vi "FTW-Actor.vi"(0 "Actor Template-Core":refnum<class "Actor Template-Core.lvclass">, 5 "FTW Actor Instance Configuration":string="{\n  \"Identity\": \"ActorName\",\n  \"InboxAddress\": \"inproc://*\",\n  \"LoggerAddress\": \"\",\n  \"My Data\": false,\n  \"Publisher URI\": \"inproc://*\",\n  \"Subscriber URIs\": \"\",\n  \"Refresh Period\": 2\n}", 11 "ErrorIn":errorcluster) -> (15 "Error":errorcluster)   [LabVIEW 2015, in "Actor Template-Core.lvclass"]
uses:
  Actor Template-Core.lvclass
  source/actor/Message/Base/FTW-Message.lvclass
  Actor Template-Core.lvclass/Actor Template-Core.ctl
  source/actor/Instance/FTW-ActorInstance.lvclass/FTW-ActorInstance.ctl
  source/actor/JobSequencer/FTW-SEQ-Current.vi
  source/actor/Connector/FTW-ActorConnector.lvclass
  source/actor/Instance/FTW-ActorInstance.lvclass
  source/actor/Message/Request/FTW-Message-IncomingRequest.lvclass
  source/actor/Publisher/FTW-Publisher.lvclass
  source/actor/Subscriber/FTW-Subscriber.lvclass
panel:
  # "#TODO\nhide controls for a GUI"
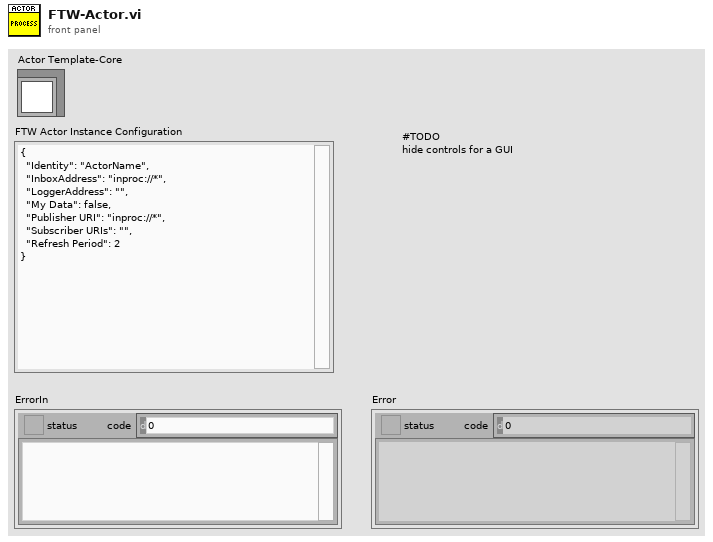
[diagram p1: front panel]
types:
  T1 = cluster{"Incoming Requests":refnum<event-registration>, "Local Messages":refnum<event-registration>, "Subscription":refnum<event-registration>}
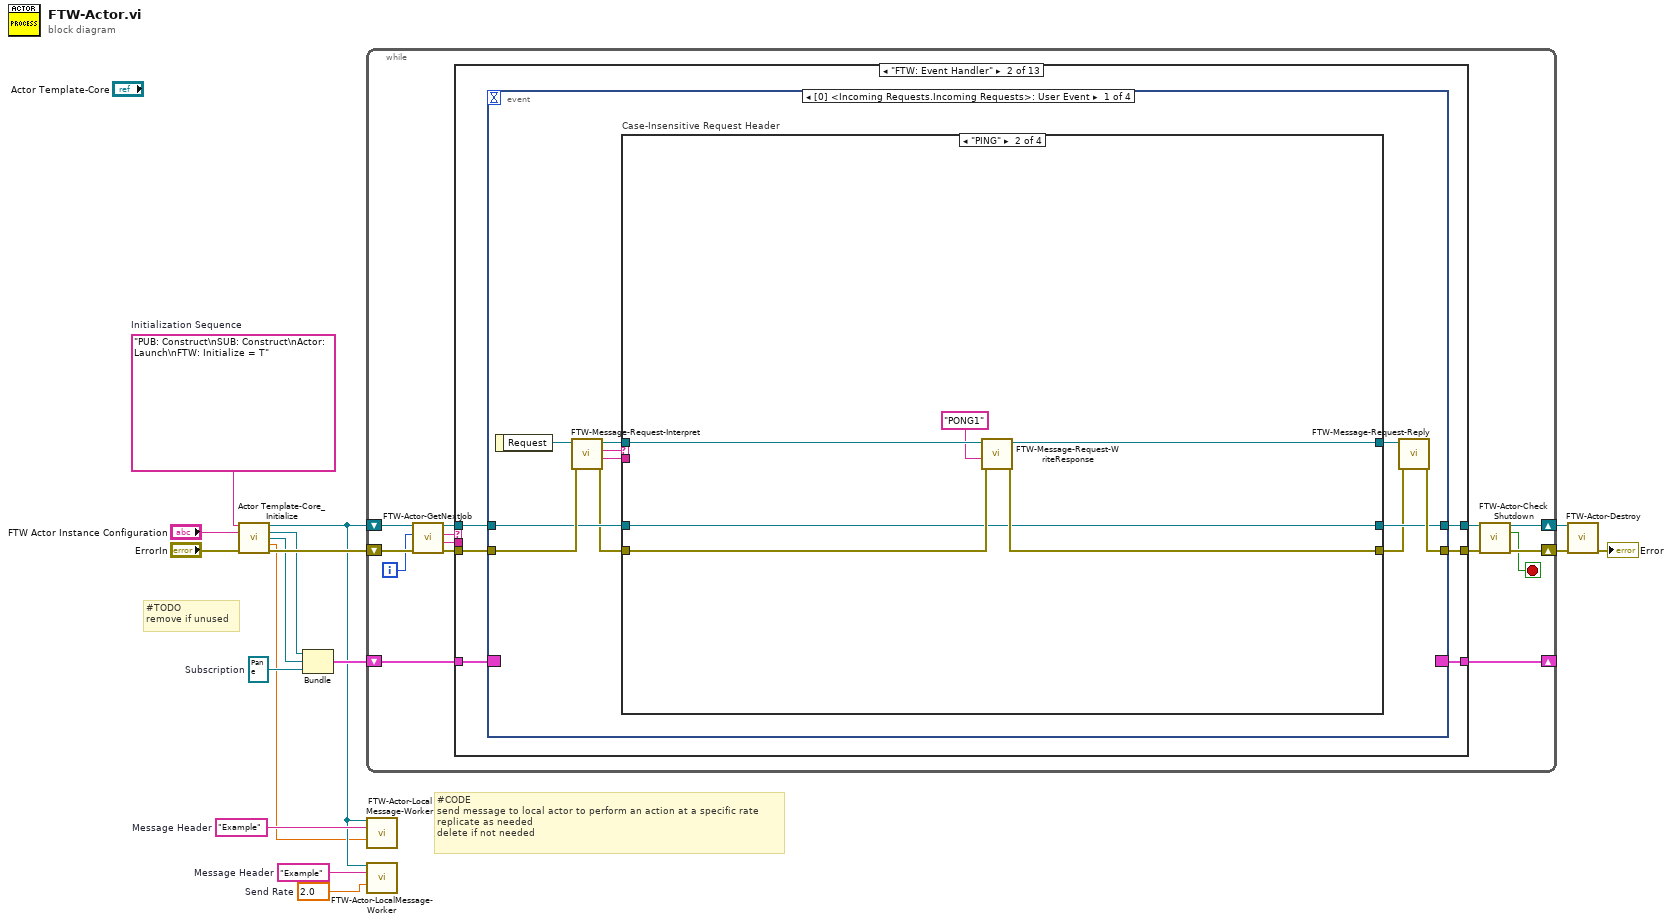
[diagram p0: block diagram]
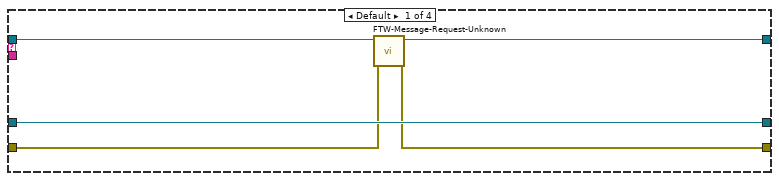
[diagram p3: hidden frame]
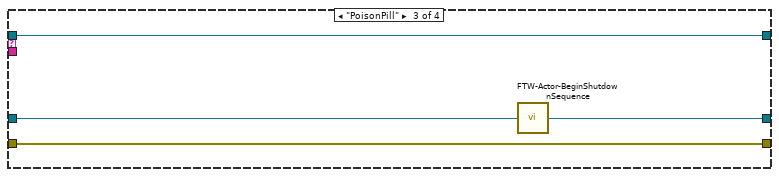
[diagram p4: hidden frame]
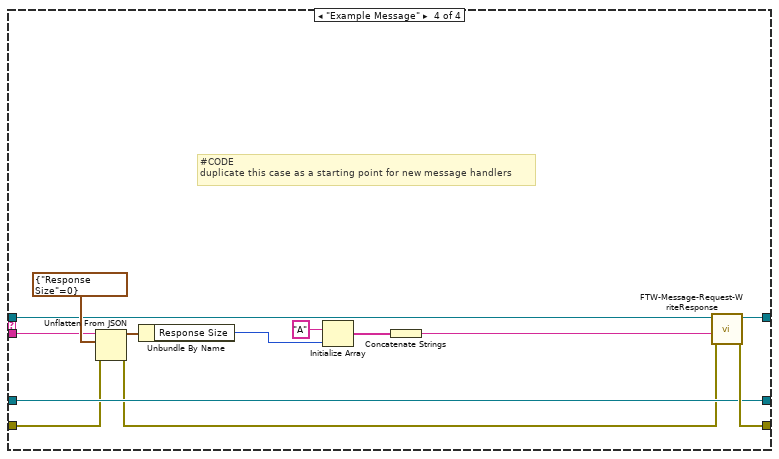
[diagram p5: hidden frame]
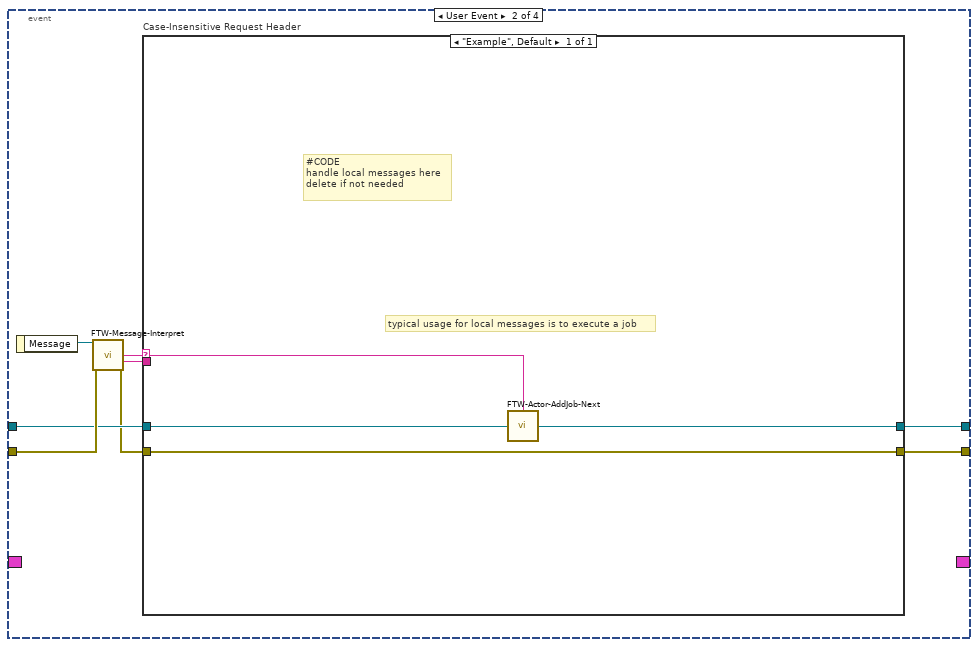
[diagram p6: hidden frame]
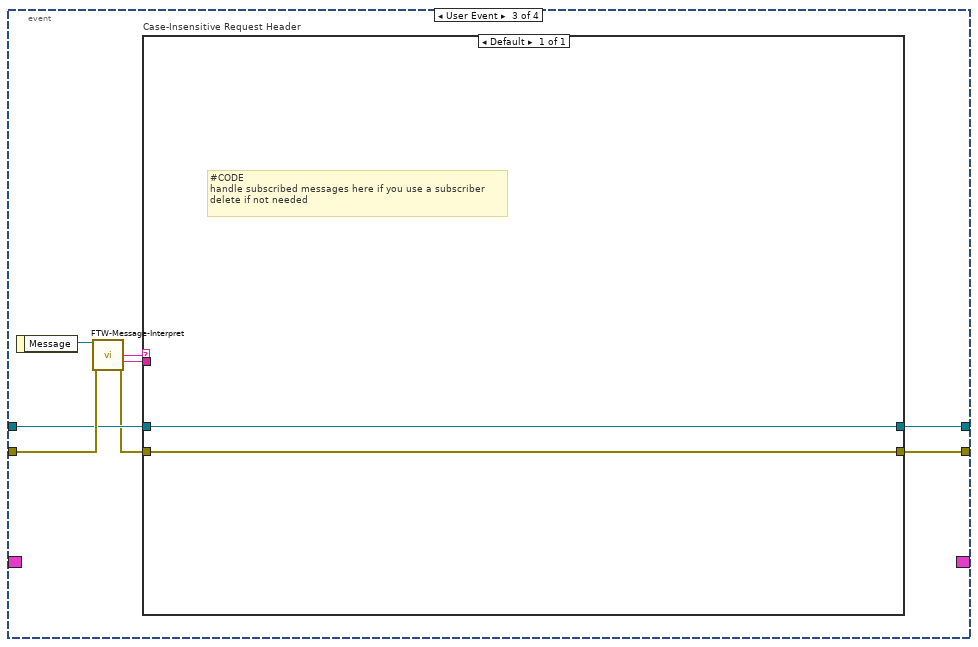
[diagram p7: hidden frame]
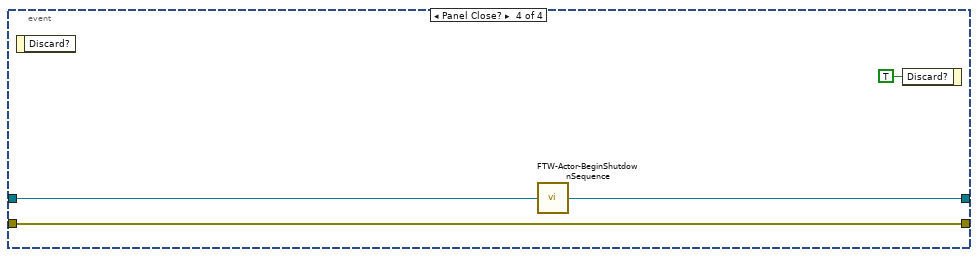
[diagram p8: hidden frame]
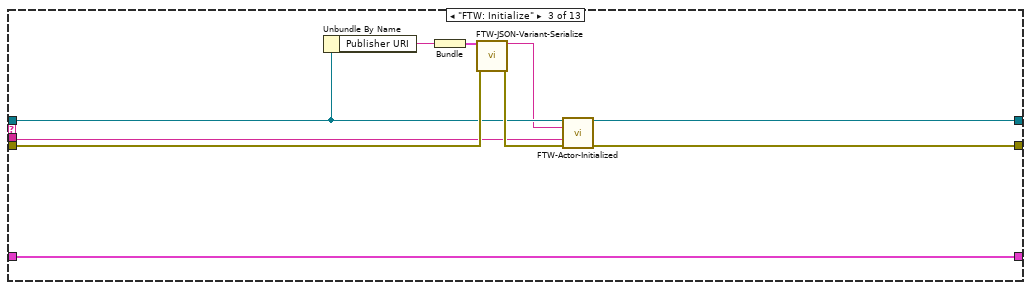
[diagram p9: hidden frame]
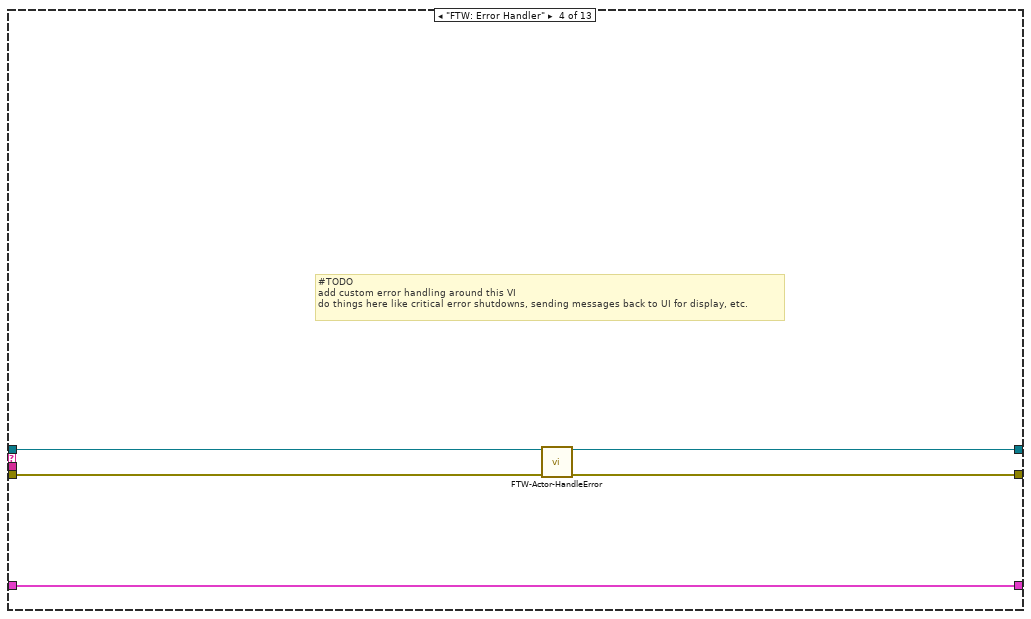
[diagram p10: hidden frame]
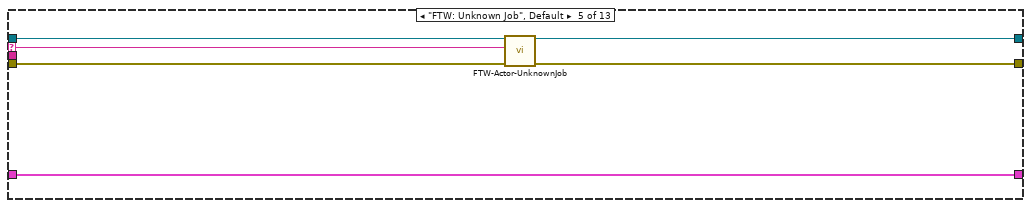
[diagram p11: hidden frame]
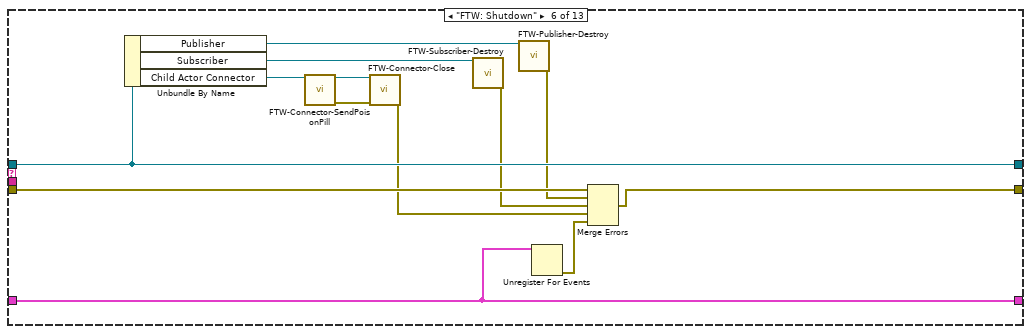
[diagram p12: hidden frame]
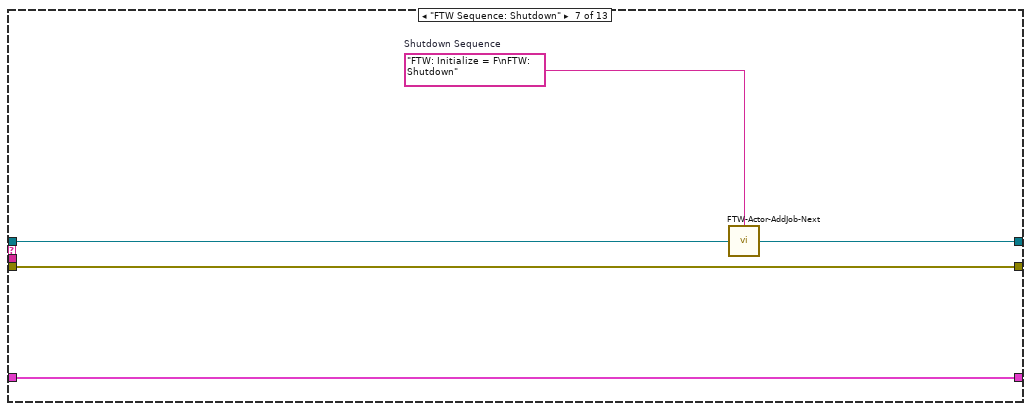
[diagram p13: hidden frame]
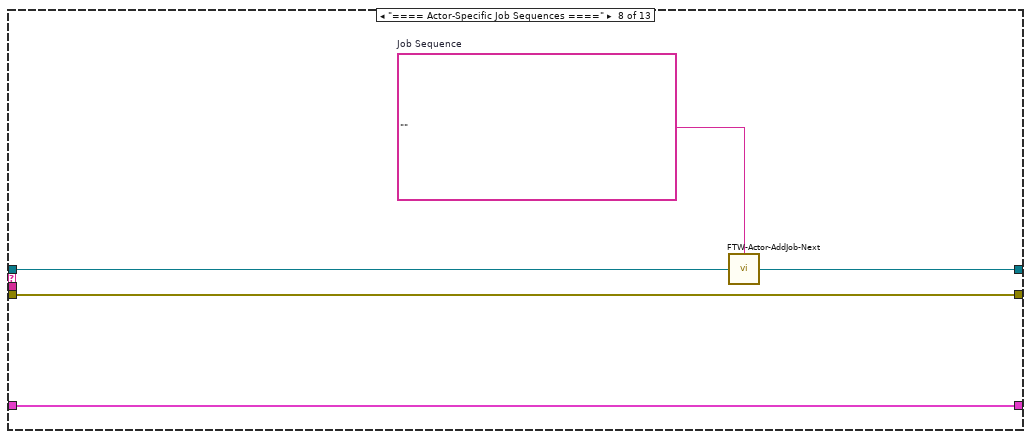
[diagram p14: hidden frame]
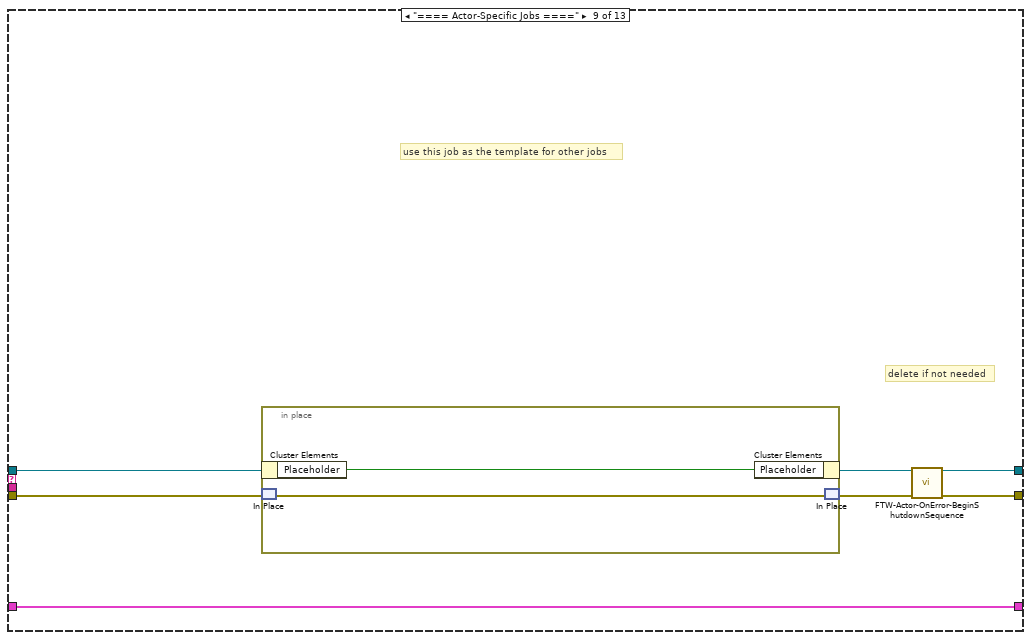
[diagram p15: hidden frame]
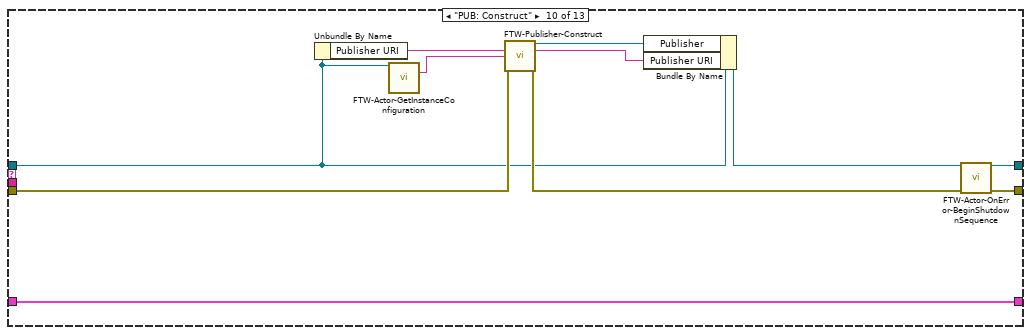
[diagram p16: hidden frame]
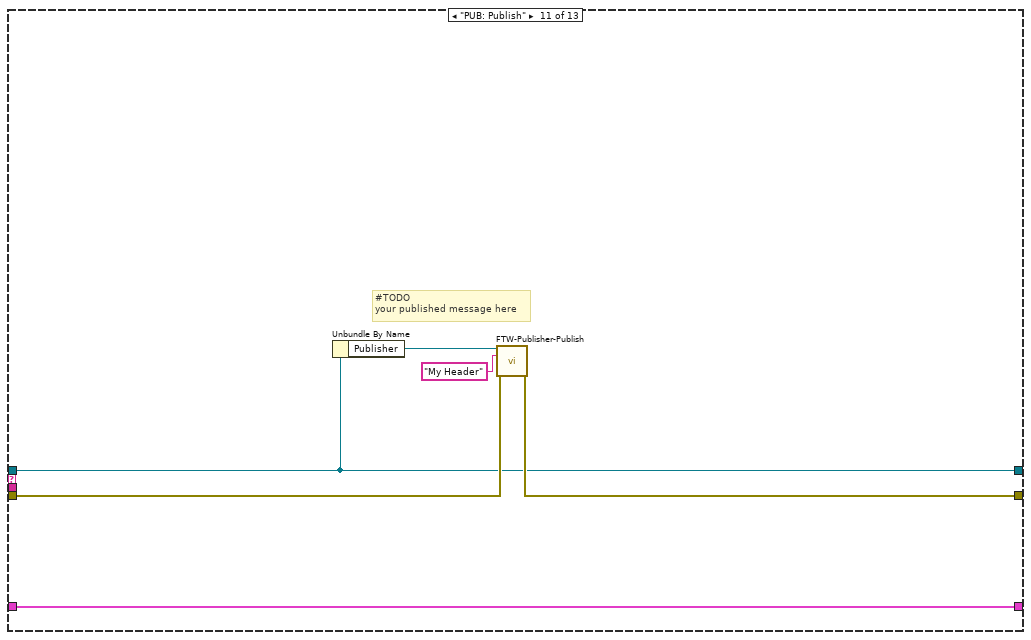
[diagram p17: hidden frame]
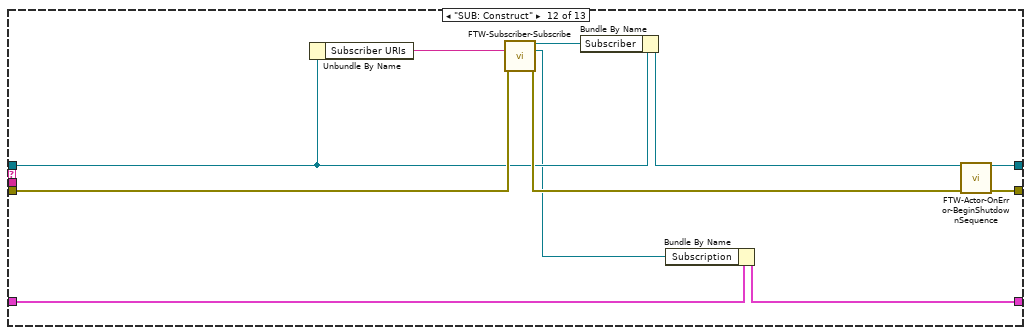
[diagram p18: hidden frame]
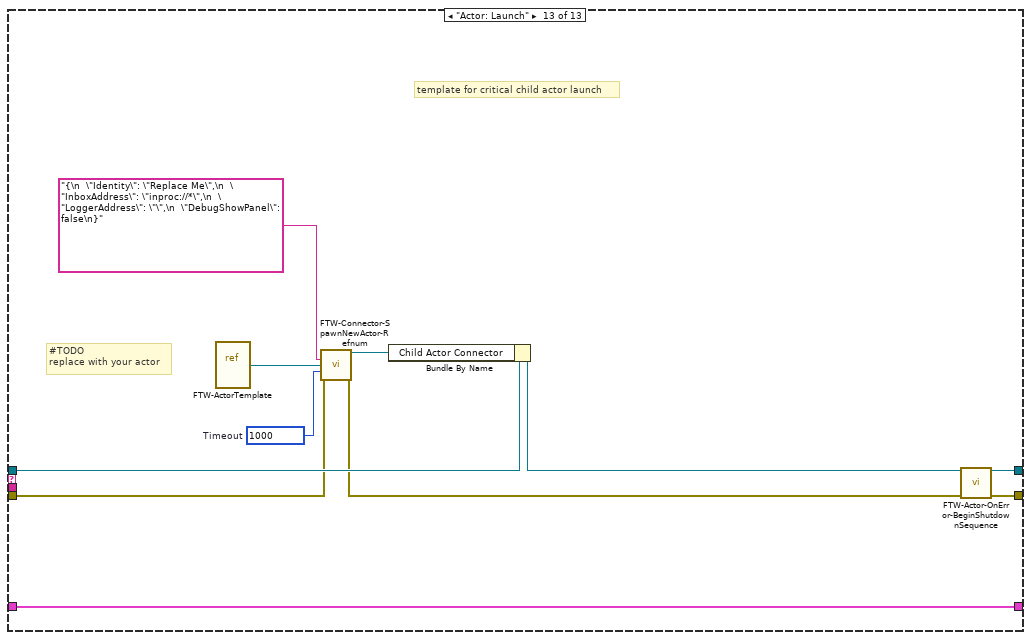
[diagram p19: hidden frame]
diagram:
  w4 = 2.0  # Send Rate
  w3 = "Example"  # Message Header
  w5 = "Example"  # Message Header
  w6 = refnum<event-registration> refnum  # Subscription
  w12 = "PUB: Construct\nSUB: Construct\nActor: Launch\nFTW: Initialize = T"  # Initialization Sequence
  # "#CODE\nsend message to local actor to perform an action at a specific rate\nreplicate as needed\ndelete if not needed"
  # "#TODO\nremove if unused"
  n1 = call "Actor Template-Core_Initialize.vi"("Initialization Sequence"=w12, "FTW Actor Instance Configuration"="FTW Actor Instance Configuration", "error in (no error)"="ErrorIn") -> ("Actor Template-Core out"=w2:refnum<class "Actor Template-Core.lvclass">, "Incoming Requests"=w8:refnum<event-registration>, "Local Messages"=w7:refnum<event-registration>, "Refresh Period"=w1:dbl, "error out"=w13:errorcluster)  [unwired: 8 in]
  n2 = Bundle("Incoming Requests"=w8, "Local Messages"=w7, "Subscription"=w6) -> (w10:T1)  [unwired: 1 in]
  n3 = while {
    shift-right: [w20] -> w15
    shift-left: w13 -> [w27]
    shift-right: [w17] -> _
    shift-left: w10 -> [w30]
    shift-right: [w22] -> w16
    shift-left: w2 -> [w29]
    i -> [w18]
    stop <- w19 stop-if-true
    n4 = call "FTW-Actor-GetNextJob.vi"("error in"=w27, "Jobs Performed"=w18, "FTW Actor Instance"=w29) -> ("error out"=w26:errorcluster, "Job Data"=w24:string, "Job Name"=w25:string, "FTW Actor Instance out"=w28:refnum<class "Actor Template-Core.lvclass">)  [unwired: 5 in]
    n5 = case shown="\"FTW: Event Handler\"" w25 {
      selector: w25 -> [_ _ _ _ w120 _ _ _ _ _ _ _ _]
      tunnel: [w32 w39 w110 w115 w123 w137 w142 w147 w151 w164 w172 w181 w195] -> w21
      tunnel: w26 -> [w32 w38 w114 w117 w124 w138 w142 w147 w154 w166 w173 w183 w189]
      tunnel: w30 -> [w33 w34 w112 w119 w125 w135 w143 w148 w155 w168 w174 w185 w196]
      tunnel: [w33 w37 w112 w119 w125 w135 w143 w148 w155 w168 w174 w176 w196] -> w17
      tunnel: w24 -> [_ _ w107 _ _ _ _ _ _ _ _ _ _]
      tunnel: [w31 w36 w111 w116 w121 w134 w140 w145 w149 w162 w171 w179 w194] -> w23
      tunnel: w28 -> [w31 w35 w109 w118 w122 w134 w141 w146 w152 w159 w171 w177 w193]
      frame "==== Featherweight Framework Jobs ====" {
      }
      frame "FTW: Event Handler" {
        n6 = event shown="[0] <Incoming Requests.Incoming Requests>: User Event" {
          selector: w34 -> [_ _ _ _]
          dyn-events: [_ _ _ _] -> w37
          timeout: _ -> [_ _ _ _]
          tunnel: [w49 w81 w93 w103] -> w39
          tunnel: w38 -> [w48 w85 w97 w103]
          tunnel: [w43 w82 w94 w101] -> w36
          tunnel: w35 -> [w47 w84 w96 w102]
          event User Event {
            n7 = event-data() -> ("Request"=w50:refnum<class "FTW-Message-IncomingRequest.lvclass">)  [unwired: 1 in]
            n8 = call "FTW-Message-Request-Interpret.vi"("error in"=w48, "FTW Incoming Request"=w50) -> ("error out"=w46:errorcluster, "Request Body"=w40:string, "Request Header"=w44:string, "FTW Incoming Request out"=w45:refnum<class "FTW-Message-IncomingRequest.lvclass">)  [unwired: 6 in]
            n9 = case "Case-Insensitive Request Header" shown="\"PING\"" w44 {
              tunnel: [w53 w59 w64 w78] -> w42
              tunnel: w46 -> [w54 w60 w64 w67]
              tunnel: [w55 w58 w65 w76] -> w43
              tunnel: w47 -> [w55 w58 w63 w76]
              tunnel: w45 -> [w52 w61 w62 w68]
              tunnel: [w51 w57 w62 w77] -> w41
              tunnel: w40 -> [_ _ _ w66]
              frame Default {
                n10 = call "FTW-Message-Request-Unknown.vi"("error in"=w54, "FTW Incoming Request"=w52) -> ("error out"=w53:errorcluster, "FTW Incoming Request Out"=w51:refnum<class "FTW-Message-IncomingRequest.lvclass">)  [unwired: 8 in]
              }
              frame "PING" {
                n11 = call "FTW-Message-Request-WriteResponse.vi"("error in"=w60, "Response Body"="PONG1" ("Response Header"), "FTW Incoming Request"=w61) -> ("error out"=w59:errorcluster, "FTW Incoming Request out"=w57:refnum<class "FTW-Message-IncomingRequest.lvclass">)  [unwired: 7 in]
              }
              frame "PoisonPill" {
                n12 = call "FTW-Actor-BeginShutdownSequence.vi"("FTW Actor Instance"=w63) -> ("FTW Actor Instance out"=w65:refnum<class "Actor Template-Core.lvclass">)  [unwired: 3 in]
              }
              frame "Example Message" {
                # "#CODE\nduplicate this case as a starting point for new message handlers"
                n13 = Unflatten From JSON(JSON string=w66, type and defaults=cluster{"Response Size":i32} {"Response Size"=0}, error in (no error)=w67) -> (value=w73:cluster{"Response Size":i32}, error out=w75:errorcluster)  [unwired: 4 in]
                n14 = Unbundle By Name(w73) -> ("Response Size"=w72:i32)
                n15 = Initialize Array("A", w72) -> (w70:string[])
                n16 = Concatenate Strings(w70) -> (w69:string)
                n17 = call "FTW-Message-Request-WriteResponse.vi"("error in"=w75, "Response Body"=w69, "FTW Incoming Request"=w68) -> ("error out"=w78:errorcluster, "FTW Incoming Request out"=w77:refnum<class "FTW-Message-IncomingRequest.lvclass">)  [unwired: 7 in]
              }
            }
            n18 = call "FTW-Message-Request-Reply.vi"("FTW: Reply Error"=w42, "FTW Incoming Request"=w41) -> ("error out"=w49:errorcluster)  [unwired: 8 in, 1 out]
          }
          event User Event {
            n19 = event-data() -> ("Message"=w86:refnum<class "FTW-Message.lvclass">)  [unwired: 1 in]
            n20 = call-dynamic "FTW-Message-Interpret.vi"("FTW Message"=w86, "error in"=w85) -> ("Message Header"=w80:string, "Message Body"=w79:string, "error out"=w83:errorcluster)  [unwired: 9 in, 2 out]
            n21 = case "Case-Insensitive Request Header" shown="\"Example\", Default" w80 {
              selector: w80 -> [w87]
              tunnel: [w89] -> w81
              tunnel: w83 -> [w89]
              tunnel: [w88] -> w82
              tunnel: w84 -> [w90]
              tunnel: w79 -> [_]
              frame "Example", Default {
                # "#CODE\nhandle local messages here\ndelete if not needed"
                # "typical usage for local messages is to execute a job"
                n22 = call "FTW-Actor-AddJob-Next.vi"("Add Next in Job Queue"=w87, "FTW Actor Instance"=w90) -> ("FTW Actor Instance out"=w88:refnum<class "Actor Template-Core.lvclass">)  [unwired: 2 in]
              }
            }
          }
          event User Event {
            n23 = event-data() -> ("Message"=w98:refnum<class "FTW-Message.lvclass">)  [unwired: 1 in]
            n24 = call-dynamic "FTW-Message-Interpret.vi"("FTW Message"=w98, "error in"=w97) -> ("Message Header"=w92:string, "Message Body"=w91:string, "error out"=w95:errorcluster)  [unwired: 9 in, 2 out]
            n25 = case "Case-Insensitive Request Header" shown="Default" w92 {
              tunnel: [w99] -> w93
              tunnel: w95 -> [w99]
              tunnel: [w100] -> w94
              tunnel: w96 -> [w100]
              tunnel: w91 -> [_]
              frame Default {
                # "#CODE\nhandle subscribed messages here if you use a subscriber\ndelete if not needed"
              }
            }
          }
          event Panel Close? {
            n26 = event-data() -> ()  [unwired: 1 in, 1 out]
            n27 = call "FTW-Actor-BeginShutdownSequence.vi"("FTW Actor Instance"=w102) -> ("FTW Actor Instance out"=w101:refnum<class "Actor Template-Core.lvclass">)  [unwired: 3 in]
            n28 = event-data("Discard?"=TRUE) -> ()  [unwired: 1 in, 1 out]
          }
        }
      }
      frame "FTW: Initialize" {
        n29 = Unbundle By Name(w109) -> ("Publisher URI"=w108:string)
        n30 = Bundle("Publisher URI"=w108) -> (w106:cluster{"Publisher URI":string})  [unwired: 1 in]
        n31 = call "FTW-JSON-Variant-Serialize.vi"("Variant"=w106, "error in"=w114) -> ("JSON String"=w105:string, "error out"=w113:errorcluster)  [unwired: 12 in]
        n32 = call-dynamic "FTW-Actor-Initialized.vi"("FTW Actor Instance"=w109, "Initialized Response"=w105, "Positive Init?"=w107, "error in"=w113) -> ("FTW Actor Instance out"=w111:refnum<class "Actor Template-Core.lvclass">, "error out"=w110:errorcluster)  [unwired: 10 in]
      }
      frame "FTW: Error Handler" {
        # "#TODO\nadd custom error handling around this VI\ndo things here like critical error shutdowns, sending messages back to UI for display, etc."
        n33 = call-dynamic "FTW-Actor-HandleError.vi"("FTW Actor Instance"=w118, "error in"=w117) -> ("FTW Actor Instance out"=w116:refnum<class "Actor Template-Core.lvclass">, "error out"=w115:errorcluster)  [unwired: 10 in, 2 out]
      }
      frame "FTW: Unknown Job", Default {
        n34 = call-dynamic "FTW-Actor-UnknownJob.vi"("FTW Actor Instance"=w122, "Unknown Job"=w120, "error in"=w124) -> ("FTW Actor Instance out"=w121:refnum<class "Actor Template-Core.lvclass">, "error out"=w123:errorcluster)  [unwired: 11 in]
      }
      frame "FTW: Shutdown" {
        n35 = Unbundle By Name(w134) -> ("Publisher"=w133:refnum<class "FTW-Publisher.lvclass">, "Subscriber"=w131:refnum<class "FTW-Subscriber.lvclass">, "Child Actor Connector"=w129:refnum<class "FTW-ActorConnector.lvclass">)
        n36 = call-dynamic "FTW-Connector-SendPoisonPill.vi"("FTW Actor Connector"=w129) -> ("FTW Actor Connector out"=w128:refnum<class "FTW-ActorConnector.lvclass">, "error out"=w127:errorcluster)  [unwired: 9 in, 4 out]
        n37 = call-dynamic "FTW-Connector-Close.vi"("FTW Actor Connector"=w128, "error in"=w127) -> ("error out"=w126:errorcluster)  [unwired: 13 in]
        n38 = call "FTW-Subscriber-Destroy.vi"("FTW-Subscription In"=w131) -> ("error out"=w130:errorcluster)  [unwired: 14 in]
        n39 = call "FTW-Publisher-Destroy.vi"("FTW-Publisher In"=w133) -> ("error out"=w132:errorcluster)  [unwired: 14 in]
        n40 = Unregister For Events(event registration refnum=w135) -> (error out=w136:errorcluster)  [unwired: 1 in]
        n41 = Merge Errors(w138, w132, w130, w126, w136) -> (w137:errorcluster)
      }
      frame "FTW Sequence: Shutdown" {
        w139 = "FTW: Initialize = F\nFTW: Shutdown"  # Shutdown Sequence
        n42 = call "FTW-Actor-AddJob-Next.vi"("Add Next in Job Queue"=w139, "FTW Actor Instance"=w141) -> ("FTW Actor Instance out"=w140:refnum<class "Actor Template-Core.lvclass">)  [unwired: 2 in]
      }
      frame "==== Actor-Specific Job Sequences ====" {
        w144 = ""  # Job Sequence
        n43 = call "FTW-Actor-AddJob-Next.vi"("Add Next in Job Queue"=w144, "FTW Actor Instance"=w146) -> ("FTW Actor Instance out"=w145:refnum<class "Actor Template-Core.lvclass">)  [unwired: 2 in]
      }
      frame "==== Actor-Specific Jobs ====" {
        # "delete if not needed"
        # "use this job as the template for other jobs"
        n44 = in-place {
          n45 = in-place-cluster #1(w152) -> ("Placeholder"=w156:bool)
          n46 = in-place-match #2(w154) -> (w157:errorcluster)
          n47 = in-place-cluster #1("Placeholder"=w156) -> (w150:refnum<class "Actor Template-Core.lvclass">)
          n48 = in-place-match #2(w157) -> (w153:errorcluster)
        }
        n49 = call-dynamic "FTW-Actor-OnError-BeginShutdownSequence.vi"("FTW Actor Instance"=w150, "error in"=w153) -> ("FTW Actor Instance out"=w149:refnum<class "Actor Template-Core.lvclass">, "error out"=w151:errorcluster)  [unwired: 12 in]
      }
      frame "PUB: Construct" {
        n50 = Unbundle By Name(w159) -> ("Publisher URI"=w160:string)
        n51 = call "FTW-Actor-GetInstanceConfiguration.vi"("FTW Actor Instance"=w159) -> ("Identity"=w158:string)  [unwired: 12 in, 2 out]
        n52 = call "FTW-Publisher-Construct.vi"("Address"=w160, "Identity"=w158, "error in"=w166) -> ("FTW-Publisher Out"=w167:refnum<class "FTW-Publisher.lvclass">, "Actual Address"=w161:string, "error out"=w165:errorcluster)  [unwired: 10 in]
        n53 = Bundle By Name(cluster=w159, "Publisher"=w167, "Publisher URI"=w161) -> (w163:refnum<class "Actor Template-Core.lvclass">)
        n54 = call-dynamic "FTW-Actor-OnError-BeginShutdownSequence.vi"("FTW Actor Instance"=w163, "error in"=w165) -> ("FTW Actor Instance out"=w162:refnum<class "Actor Template-Core.lvclass">, "error out"=w164:errorcluster)  [unwired: 12 in]
      }
      frame "PUB: Publish" {
        # "#TODO\nyour published message here"
        n55 = Unbundle By Name(w171) -> ("Publisher"=w170:refnum<class "FTW-Publisher.lvclass">)
        n56 = call "FTW-Publisher-Publish.vi"("FTW-Publisher In"=w170, "Header"="My Header", "error in"=w173) -> ("error out"=w172:errorcluster)  [unwired: 11 in, 1 out]
      }
      frame "SUB: Construct" {
        n57 = Unbundle By Name(w177) -> ("Subscriber URIs"=w178:string)
        n58 = call "FTW-Subscriber-Subscribe.vi"("Addresses"=w178, "error in"=w183) -> ("FTW-Subscription Out"=w184:refnum<class "FTW-Subscriber.lvclass">, "Subscriber Registration"=w175:refnum<event-registration>, "error out"=w182:errorcluster)  [unwired: 11 in]
        n59 = Bundle By Name(cluster=w177, "Subscriber"=w184) -> (w180:refnum<class "Actor Template-Core.lvclass">)
        n60 = Bundle By Name(cluster=w185, "Subscription"=w175) -> (w176:T1)
        n61 = call-dynamic "FTW-Actor-OnError-BeginShutdownSequence.vi"("FTW Actor Instance"=w180, "error in"=w182) -> ("FTW Actor Instance out"=w179:refnum<class "Actor Template-Core.lvclass">, "error out"=w181:errorcluster)  [unwired: 12 in]
      }
      frame "Actor: Launch" {
        w192 = 1000  # Timeout
        # "#TODO\nreplace with your actor"
        # "template for critical child actor launch"
        n62 = vi-ref "FTW-ActorTemplate.vi"() -> (w191:refnum<vi>)
        n63 = call "FTW-Connector-SpawnNewActor-Refnum.vi"("Configuration"="{\n  \"Identity\": \"Replace Me\",\n  \"InboxAddress\": \"inproc://*\",\n  \"LoggerAddress\": \"\",\n  \"DebugShowPanel\": false\n}", "Actor VI Refnum"=w191, "Timeout"=w192, "error in"=w189) -> ("FTW Actor Connector"=w186:refnum<class "FTW-ActorConnector.lvclass">, "error out"=w188:errorcluster)  [unwired: 8 in, 2 out]
        n64 = Bundle By Name(cluster=w193, "Child Actor Connector"=w186) -> (w187:refnum<class "Actor Template-Core.lvclass">)
        n65 = call-dynamic "FTW-Actor-OnError-BeginShutdownSequence.vi"("FTW Actor Instance"=w187, "error in"=w188) -> ("FTW Actor Instance out"=w194:refnum<class "Actor Template-Core.lvclass">, "error out"=w195:errorcluster)  [unwired: 12 in]
      }
    }
    n66 = call "FTW-Actor-CheckShutdown.vi"("FTW Actor Instance"=w23, "error in"=w21) -> ("FTW Actor Instance out"=w22:refnum<class "Actor Template-Core.lvclass">, "Shutdown?"=w19:bool, "error out"=w20:errorcluster)  [unwired: 11 in]
  }
  n67 = call-dynamic "FTW-Actor-LocalMessage-Worker.vi"("FTW-ActorInstance In"=w2, "Message Header"=w5, "Send Rate"=w1) -> ()  [unwired: 13 in]
  n68 = call-dynamic "FTW-Actor-LocalMessage-Worker.vi"("FTW-ActorInstance In"=w2, "Message Header"=w3, "Send Rate"=w4) -> ()  [unwired: 13 in]
  n69 = call-dynamic "FTW-Actor-Destroy.vi"("FTW Actor Instance"=w16, "error in"=w15) -> ("error out"=→"Error":errorcluster)  [unwired: 13 in]
